vi "Subscribe Client.vi"(8 "error in":errorcluster, 9 "Client":string, 10 "Topic Name":string, 11 "Broker in":refnum<class "Broker.lvclass">) -> (0 "error out":errorcluster, 3 "Broker out":refnum<class "Broker.lvclass">)   [LabVIEW 2014, in "Broker.lvclass"]
uses:
  Broker.lvclass
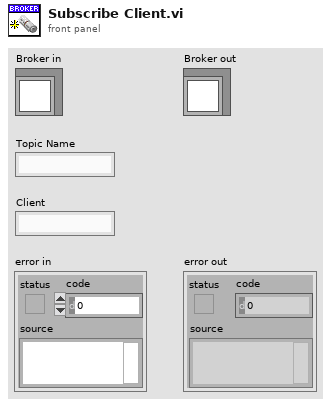
[diagram p1: front panel]
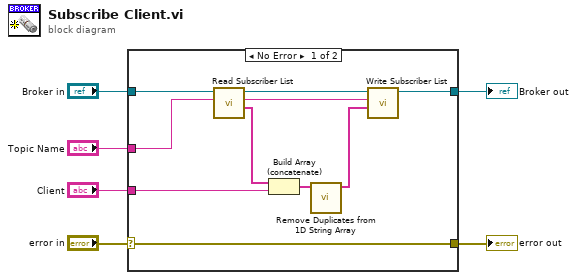
[diagram p0: block diagram]
diagram:
  n1 = case shown="No Error" "error in" {
    selector: "error in" -> [w15 w18]
    tunnel: [w15 w18] -> w5
    tunnel: [w13 w17] -> w3
    tunnel: "Broker in" -> [w16 w17]
    tunnel: "Client" -> [w11 _]
    tunnel: "Topic Name" -> [w7 _]
    frame No Error {
      n2 = call-dynamic "Read Subscriber List.vi"("Topic Name"=w7, "Broker in"=w16) -> ("Subscriber List"=w12:string[], "Topic Name Out"=w8:string, "Broker out"=w14:refnum<class "Broker.lvclass">)  [unwired: 6 in, 1 out]
      n3 = Build Array (concatenate)(w12, w11) -> (w10:string[])
      n4 = call "Remove Duplicates from 1D String Array.vi"("Input Array"=w10) -> ("Output Array"=w9:string[])  [unwired: 10 in]
      n5 = call-dynamic "Write Subscriber List.vi"("Subscriber List"=w9, "Topic Name"=w8, "Broker in"=w14) -> ("Broker out"=w13:refnum<class "Broker.lvclass">)  [unwired: 7 in, 1 out]
    }
    frame Error {
    }
  }
  "error out" <- w5
  "Broker out" <- w3
